vi "CLD 11 Producer consumer events front panel.vi"() -> ()   [LabVIEW 2015]
doc: "CLD 11 exercise"
uses:
  CLD 11 CSV file enum.ctl
panel:
  out "Current Time target":dbl
  out "Step 3":bool
  out "Step 2":bool
  out "Step 1":bool
  out "Time Has Elapsed":bool
  out "Elapsed Time":string
  in  "Auto Reset":bool=TRUE
  in  "Reset Button":bool
  in  "Stop VI":bool
  in  "Time Target (s)":dbl
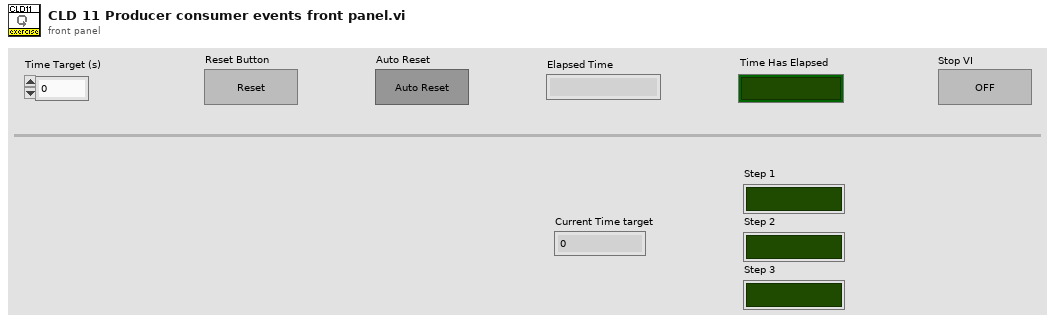
[diagram p1: front panel]
types:
  T1 = typedef "CLD 11 CSV file enum.ctl" = enum16{"Read CSV", "Write CSV"}
  T2 = typedef "CLD 11 CSV file data structure.ctl" = cluster{"Dwell Time":i32, "State 1":bool, "State 2":bool, "State 3":bool}
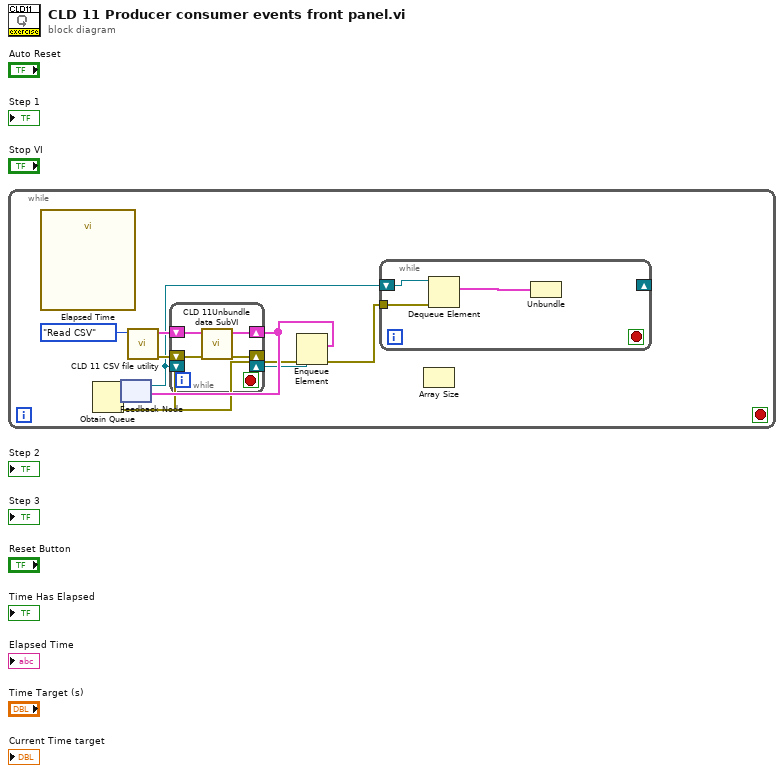
[diagram p0: block diagram]
diagram:
  n1 = while {
    stop <- _ stop-if-true
    n2 = call "Elapsed Time"() -> ()  [unwired: 12 in, 8 out]
    n3 = feedback #1() -> (w2:refnum<queue>)  [unwired: 1 in]
    n4 = call "CLD 11 CSV file utility.vi"("CSV File Enum"=CLD_11_CSV_file_enum."Read CSV") -> ("Error Out"=w5:errorcluster, "[Data Out]"=w9:T2[])  [unwired: 9 in]
    n5 = while {
      shift-right: [w16] -> w8
      shift-left: w9 -> [w17]
      shift-right: [w15] -> w6
      shift-left: w5 -> [w14]
      shift-right: [_] -> w3
      shift-left: w2 -> [_]
      stop <- _ stop-if-true
      n6 = call "CLD 11Unbundle data SubVI.vi"("error in (no error)"=w14, "[Data In]"=w17) -> ("error out"=w15:errorcluster, "[Data Out]"=w16:T2[])  [unwired: 3 in, 5 out]
    }
    n7 = Obtain Queue(element data type=w8, error in (no error)=w6) -> (queue out=w4:refnum<queue>, error out=w7:errorcluster)  [unwired: 3 in, 1 out]
    n8 = feedback-in #1(w4) -> ()
    n9 = Enqueue Element(queue=w3, element=w8, error in (no error)=w7) -> (error out=w1:errorcluster)  [unwired: 1 in, 2 out]
    n10 = while {
      shift-right: _ -> [_]
      shift-left: w2 -> [w13]
      tunnel: w1 -> [w12]
      stop <- _ stop-if-true
      n11 = Dequeue Element(queue=w13, error in (no error)=w12) -> (element=w11:T2[])  [unwired: 1 in, 3 out]
      n12 = Unbundle(w11) -> ()  [unwired: 2 out]
    }
    n13 = Array Size() -> ()  [unwired: 1 in, 1 out]
  }
